vi "Ultrasonic Init.vi"(8 "error in (no error)":errorcluster) -> (0 "error out":errorcluster, 3 "Ultrasonic":T1)   [LabVIEW 2020]
uses:
  <vilib>/High Genius/HG_WSI_Tookit/Dependencies/Library/Pulse/Pulse.lvclass
  C:/Program Files (x86)/National Instruments/LabVIEW 2020/vi.lib/High Genius/HG_WSI_Tookit/Dependencies/Library/HG_LIB/HG_LIB.lvclass
  <vilib>/High Genius/HG_WSI_Tookit/Dependencies/Library/ISQ/ISQ.lvclass
  <vilib>/High Genius/HG_WSI_Tookit/Dependencies/Library/HG_LIB/HG_LIB.lvclass
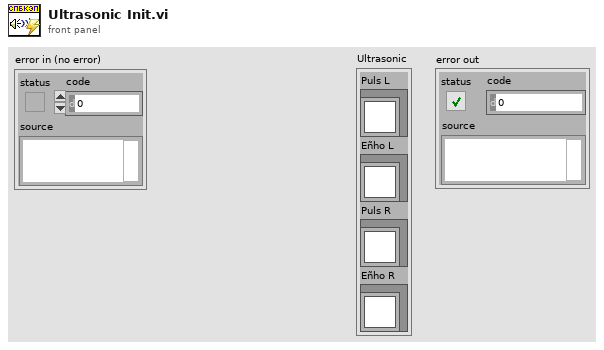
[diagram p1: front panel]
types:
  T1 = cluster{"Puls L":refnum<class "Pulse.lvclass">, "Eñho L":refnum<class "ISQ.lvclass">, "Puls R":refnum<class "Pulse.lvclass">, "Eñho R":refnum<class "ISQ.lvclass">}
  T2 = enum16{"DI", "DO", "AI", "Pulse", "PWM", "ISQ", "ENC", "CAN", "IIC", "IMU"}
  T3 = enum16{"0", "1", "2", "3", "4", "5", "6", "7", "8", "9", "10", "11", "12", "13", "14", "15", "16", "17", "18", "19", "20", "21", "22", "23", "24", "25"}
  T4 = cluster{"HG_LIB out":refnum<class "Pulse.lvclass">, "HG_LIB out":refnum<class "ISQ.lvclass">, "HG_LIB out":refnum<class "Pulse.lvclass">, "HG_LIB out":refnum<class "ISQ.lvclass">}
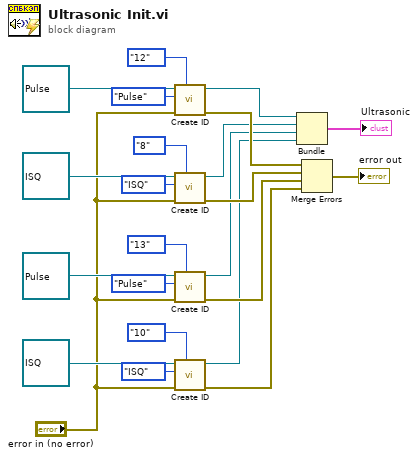
[diagram p0: block diagram]
diagram:
  n1 = call <vilib>:"Create ID.vi"("NO"=T3."12", "error in (no error)"="error in (no error)", "Function"=T2."Pulse", "HG_LIB in"=refnum<class "Pulse.lvclass"> refnum ("VMX Library.lvlib:Pulse.lvclass")) -> ("error out"=w8:errorcluster, "HG_LIB out"=w7:refnum<class "Pulse.lvclass">)  [unwired: 6 in]
  n2 = call <vilib>:"Create ID.vi"("NO"=T3."8", "error in (no error)"="error in (no error)", "Function"=T2."ISQ", "HG_LIB in"=refnum<class "ISQ.lvclass"> refnum ("ISQ.lvclass")) -> ("error out"=w9:errorcluster, "HG_LIB out"=w6:refnum<class "ISQ.lvclass">)  [unwired: 6 in]
  n3 = call <vilib>:"Create ID.vi"("NO"=T3."13", "error in (no error)"="error in (no error)", "Function"=T2."Pulse", "HG_LIB in"=refnum<class "Pulse.lvclass"> refnum ("VMX Library.lvlib:Pulse.lvclass")) -> ("error out"=w10:errorcluster, "HG_LIB out"=w5:refnum<class "Pulse.lvclass">)  [unwired: 6 in]
  n4 = call <vilib>:"Create ID.vi"("NO"=T3."10", "error in (no error)"="error in (no error)", "Function"=T2."ISQ", "HG_LIB in"=refnum<class "ISQ.lvclass"> refnum ("ISQ.lvclass")) -> ("error out"=w11:errorcluster, "HG_LIB out"=w4:refnum<class "ISQ.lvclass">)  [unwired: 6 in]
  n5 = Bundle("HG_LIB out"=w7, "HG_LIB out"=w6, "HG_LIB out"=w5, "HG_LIB out"=w4) -> (→"Ultrasonic":T4)  [unwired: 1 in]
  n6 = Merge Errors(w8, w9, w10, w11) -> (→"error out":errorcluster)
